vi "AlternatingLEDs.vi"() -> ()   [LabVIEW 2014]
panel:
  in  "stop":bool
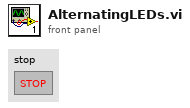
[diagram p1: front panel]
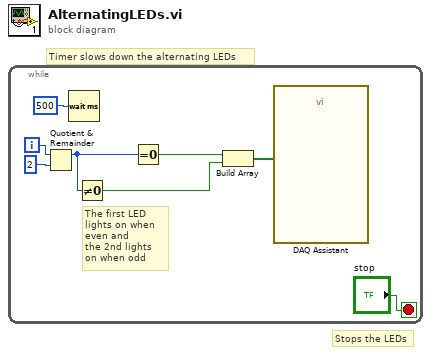
[diagram p0: block diagram]
diagram:
  # "Stops the LEDs"
  # "Timer slows down the alternating LEDs"
  n1 = while {
    i -> [w7]
    stop <- "stop" stop-if-true
    # "The first LED lights on when even and \nthe 2nd lights on when odd"
    n2 = Quotient & Remainder(x=w7, y=2) -> (x-y*floor(x/y)=w5:i32)  [unwired: 1 out]
    n3 = Wait (ms)(milliseconds to wait=500) -> ()  [unwired: 1 out]
    n4 = Not Equal To 0?(x=w5) -> (x != 0?=w2:bool)
    n5 = Equal To 0?(x=w5) -> (x = 0?=w1:bool)
    n6 = Build Array(w1, w2) -> (w8:bool[])
    n7 = call "DAQ Assistant"("data"=w8) -> ()  [unwired: 17 in, 2 out]
  }
